vi "DemoWriteDigital.vi"() -> ()   [LabVIEW 2009]
uses:
  <vilib>/NXT/Block Support/NXT_InputPort.ctl
  <vilib>/NXT/Dual Mode Library/Waits/Wait_Num(msec).vi
panel:
  in  "stop":bool
  # "Demo Digital Write"
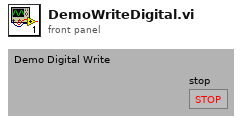
[diagram p1: front panel]
types:
  T1 = typedef "NXT_InputPort.ctl" = u8
  T2 = typedef "LVHSConnector.ctl" = cluster{"error":errorcluster, "address":string, "NXT #":i32, "Show Error":bool, "Connection":u16}
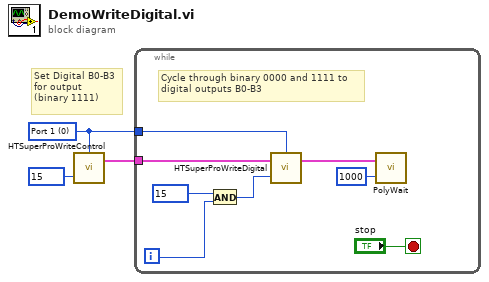
[diagram p0: block diagram]
diagram:
  w2 = T1 0 items=["Port 1", "Port 2", "Port 3", "Port 4"] ("Port")
  # "Set Digital B0-B3\nfor output\n(binary 1111)"
  n1 = call "HTSuperProWriteControl.vi"("Digital Control"=u8 15, "Port"=w2) -> ("NXT"=w3:T2)  [unwired: 3 in]
  n2 = while {
    tunnel: w3 -> [w9]
    tunnel: w2 -> [w8]
    i -> [w7]
    stop <- "stop" stop-if-true
    # "Cycle through binary 0000 and 1111 to\ndigital outputs B0-B3"
    n3 = And(x=u8 15 ("Digital Control"), y=w7) -> (x .and. y?=w5:i32)
    n4 = call "HTSuperProWriteDigital.vi"("Digital Value"=w5, "NXT"=w9, "Port"=w8) -> ("NXT"=w4:T2)  [unwired: 2 in]
    n5 = call-poly <vilib>:"PolyWait.vi"("Time (100 msec)"=u32 1000, "NXT"=w4) -> ()  [unwired: 2 in, 1 out]
  }
